vi "CalculateDeltaS.vi"(11 "Circle time series":dbl[][](array[numeric])) -> (3 "Pupil Displacement":dbl)   [LabVIEW 2013]
doc: "Returns the displacement of the pupil between the last two frames"
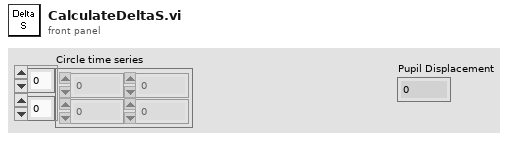
[diagram p1: front panel]
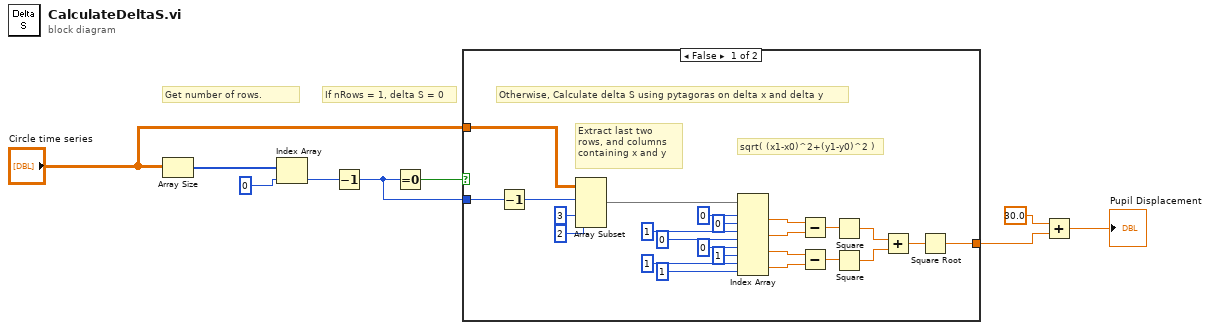
[diagram p0: block diagram]
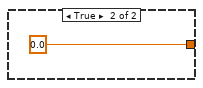
[diagram p2: hidden frame]
diagram:
  # "If nRows = 1, delta S = 0"
  # "Get number of rows."
  n1 = Array Size(array="Circle time series") -> (size(s)=w4:i32[])
  n2 = Index Array(array=w4, index=0) -> (element=w6:i32)
  n3 = Decrement(x=w6) -> (x-1=w9:i32)
  n4 = Equal To 0?(x=w9) -> (x = 0?=w7:bool)
  n5 = case shown="False" w7 {
    tunnel: "Circle time series" -> [w33 _]
    tunnel: w9 -> [w32 _]
    tunnel: [w24 0.0] -> w3
    frame False {
      # "sqrt( (x1-x0)^2+(y1-y0)^2 )"
      # "Extract last two rows, and columns containing x and y"
      # "Otherwise, Calculate delta S using pytagoras on delta x and delta y"
      n6 = Decrement(x=w32) -> (x-1=w31:i32)
      n7 = Array Subset(array=w33, index (row)=w31, index (col)=3 ("index"), length (col)=2 ("length")) -> (w25:dbl[][])  [unwired: 1 in]
      n8 = Index Array(array=w25, index (row) #1=0 ("index (row)"), index (col) #1=0 ("disabled index (col)"), index (row) #2=1 ("index (row)"), index (col) #2=0 ("disabled index (col)"), index (row) #3=0 ("index (row)"), index (col) #3=1 ("disabled index (col)"), index (row) #4=1 ("index (row)"), index (col) #4=1 ("disabled index (col)")) -> (element #1=w15:dbl, element #2=w14:dbl, element #3=w12:dbl, element #4=w11:dbl)
      n9 = Subtract(x=w15, y=w14) -> (x-y=w13:dbl)
      n10 = Subtract(x=w12, y=w11) -> (x-y=w10:dbl)
      n11 = Square(x=w13) -> (x^2=w28:dbl)
      n12 = Square(x=w10) -> (x^2=w27:dbl)
      n13 = Add(x=w28, y=w27) -> (x+y=w26:dbl)
      n14 = Square Root(x=w26) -> (sqrt(x)=w24:dbl)
    }
    frame True {
    }
  }
  n15 = Add(x=30.0, y=w3) -> (x+y=→"Pupil Displacement":dbl)
